vi "Close_ExcelApp.vi"(2 "错误输入（无错误）":errorcluster, 3 "application引用":refnum<k7>) -> (0 "错误输出":errorcluster)   [LabVIEW 2014]
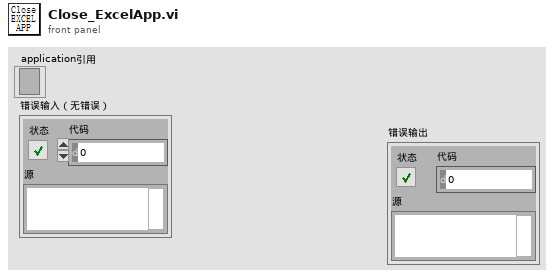
[diagram p1: front panel]
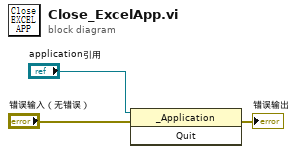
[diagram p0: block diagram]
diagram:
  n1 = invoke class="_Application" method="Quit"(reference="application引用", error in="错误输入（无错误）") -> (error out=→"错误输出":errorcluster)  [unwired: 1 in, 2 out]
